vi "InsertVariableMenuBuild.vi"(8 "error in (no error)":errorcluster, 9 "Insert Tag":string="USERVAR_TOP", 10 "menu reference in":refnum<k9>, 11 "VariableManager Ref in":refnum<vi>) -> (0 "error out":errorcluster, 2 "menu reference out":refnum<k9>)   [LabVIEW 2013]
uses:
  VariableManagerCodes/VariableManager/VariableManager.lvclass
  <vilib>/Utility/error.llb/DialogType.ctl
  VariableManagerCodes/Variable/Variable.lvclass
  VariableManagerCodes/VariableGroup/VariableGroup.lvclass
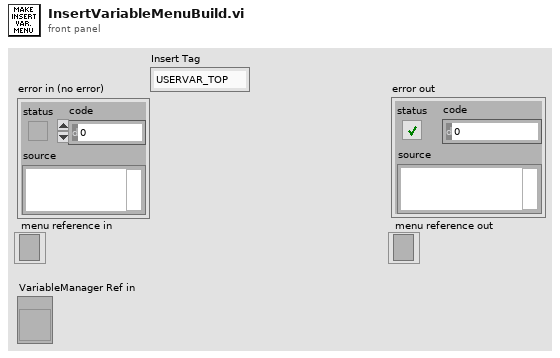
[diagram p1: front panel]
types:
  T1 = typedef "DialogType.ctl" = u16
  T2 = cluster{"MenuName":string, "MenuTag":string, "VariableNames":string[], "VariableTags":string[]}
  T3 = cluster{"MenuName":string, "MenuTag":string, "VariableNames":string[], "VariableTags":string[]}[]
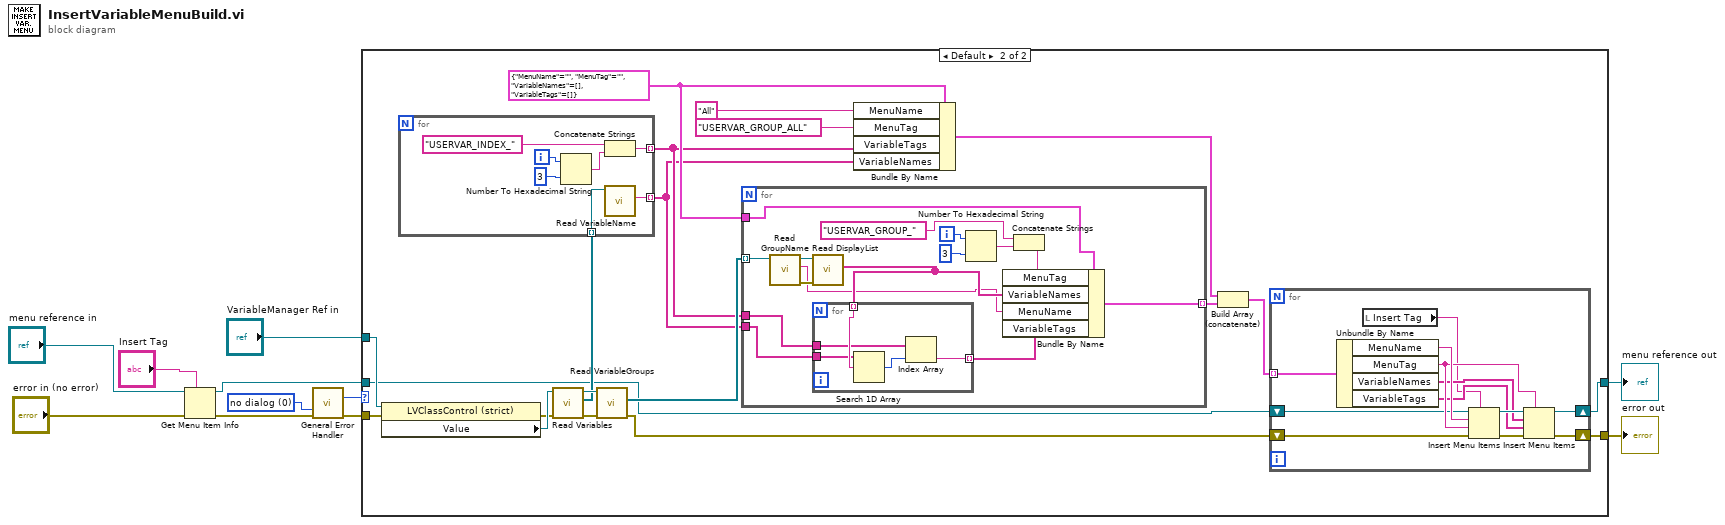
[diagram p0: block diagram]
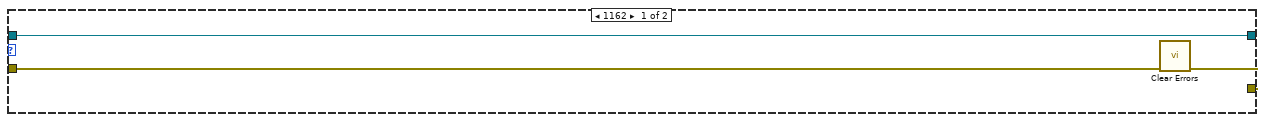
[diagram p2: hidden frame]
diagram:
  w7 = T1 0 items=["no dialog", "OK message", "continue or stop message", "OK message + warnings", "continue/stop + warnings"] ("type of dialog (OK msg:1)")
  n1 = Get Menu Item Info(7:"Insert Tag", 8:"error in (no error)", 11:"menu reference in") -> (0:w8:errorcluster, 3:w2:refnum<k9>)  [unwired: 5 out]
  n2 = call <vilib>:"General Error Handler.vi"("type of dialog (OK msg:1)"=w7, "error in (no error)"=w8) -> ("code out"=w5:i32, "error out"=w1:errorcluster)  [unwired: 9 in, 3 out]
  n3 = case shown="Default" w5 {
    tunnel: [w13 w21] -> w11
    tunnel: [w12 w20] -> w10
    tunnel: "VariableManager Ref in" -> [_ w19]
    tunnel: w1 -> [w14 w17]
    tunnel: w2 -> [w12 w15]
    frame 1162 {
      n4 = call <vilib>:"Clear Errors.vi"("error in (no error)"=w14) -> ("error out"=w13:errorcluster)  [unwired: 6 in]
    }
    frame Default {
      w30 = T2 {"MenuName"="", "MenuTag"="", "VariableNames"=[], "VariableTags"=[]} ("input cluster")
      n5 = property class="LVClassControl (strict)"(reference=w19, error in=w17) -> (error out=w16:errorcluster, "Value"=w18:refnum<class "VariableManager.lvclass">)  [unwired: 1 out]
      n6 = call-dynamic "Read Variables.vi"("error in (no error)"=w16, "VariableManager in"=w18) -> ("error out"=w33:errorcluster, "Variables"=w31:refnum<class "Variable.lvclass">[], "VariableManager out"=w34:refnum<class "VariableManager.lvclass">)  [unwired: 7 in]
      n7 = for {
        tunnel: w31 -> [w53] mode=indexing
        tunnel: [w48] -> w26 mode=indexing
        tunnel: [w47] -> w27 mode=indexing
        i -> [w50]
        n8 = Number To Hexadecimal String(1:i16 3 ("width (-)"), 2:w50) -> (0:w52:string)
        n9 = Concatenate Strings("USERVAR_INDEX_" ("initial string"), w52) -> (w47:string)
        n10 = call-dynamic "Read VariableName.vi"("Variable in"=w53) -> ("VariableName"=w48:string)  [unwired: 8 in, 2 out]
      }
      n11 = call-dynamic "Read VariableGroups.vi"("error in (no error)"=w33, "VariableManager in"=w34) -> ("error out"=w22:errorcluster, "VariableGroups"=w32:refnum<class "VariableGroup.lvclass">[])  [unwired: 7 in, 1 out]
      n12 = for {
        tunnel: w32 -> [w68] mode=indexing
        tunnel: w26 -> [w61]
        tunnel: w27 -> [w60]
        tunnel: [w58] -> w24 mode=indexing
        tunnel: w30 -> [w57]
        i -> [w66]
        n13 = call-dynamic "Read GroupName.vi"("VariableGroup in"=w68) -> ("error out"=w63:errorcluster, "GroupName"=w54:string, "VariableGroup out"=w62:refnum<class "VariableGroup.lvclass">)  [unwired: 8 in]
        n14 = call-dynamic "Read DisplayList.vi"("error in (no error)"=w63, "VariableGroup in"=w62) -> ("DisplayList"=w55:string[])  [unwired: 7 in, 2 out]
        n15 = for {
          tunnel: w55 -> [w73] mode=indexing
          tunnel: w61 -> [w72]
          tunnel: w60 -> [w70]
          tunnel: [w69] -> w59 mode=indexing
          n16 = Search 1D Array(1D array=w72, element=w73) -> (index of element=w71:i32)  [unwired: 1 in]
          n17 = Index Array(array=w70, index=w71) -> (element=w69:string)
        }
        n18 = Number To Hexadecimal String(1:i16 3 ("width (-)"), 2:w66) -> (0:w64:string)
        n19 = Concatenate Strings("USERVAR_GROUP_" ("initial string"), w64) -> (w56:string)
        n20 = Bundle By Name(cluster=w57, "MenuTag"=w56, "VariableNames"=w55, "MenuName"=w54, "VariableTags"=w59) -> (w58:T2)
      }
      n21 = Bundle By Name(cluster=w30, "MenuName"="All", "MenuTag"="USERVAR_GROUP_ALL", "VariableTags"=w27, "VariableNames"=w26) -> (w25:T2)
      n22 = Build Array (concatenate)(w25, w24) -> (w23:T3)
      n23 = for {
        tunnel: w23 -> [w44] mode=indexing
        shift-right: [w46] -> w20
        shift-left: w15 -> [w36]
        shift-right: [w45] -> w21
        shift-left: w22 -> [w35]
        n24 = Unbundle By Name(w44) -> ("MenuName"=w41:string, "MenuTag"=w40:string, "VariableNames"=w39:string[], "VariableTags"=w38:string[])
        n25 = local read "Insert Tag"() -> (w37:string)
        n26 = Insert Menu Items(5:w37, 6:w35, 7:w40, 8:w41, 9:w36) -> (0:w43:errorcluster, 3:w42:refnum<k9>)  [unwired: 1 in, 1 out]
        n27 = Insert Menu Items(5:w40, 6:w43, 7:w38, 8:w39, 9:w42) -> (0:w45:errorcluster, 3:w46:refnum<k9>)  [unwired: 1 in, 1 out]
      }
    }
  }
  "error out" <- w11
  "menu reference out" <- w10
